vi "quick_plot_for_one_channel.vi"() -> ()   [LabVIEW 2018]
uses:
  <vilib>/Utility/file.llb/Read Delimited Spreadsheet (string).vi
panel:
  in  "End Time":timestamp
  in  "Start Time":timestamp
  in  "Property":T1(ring)
  out "Graph":cluster{timestamp[], dbl[]}(graph)
  out "all rows":string[][](array[string])
  # "As of 16-01-2020 columns are:\n[0]: on/off\n[1]: status\n[2]: channel name\n[3]: crate\n[4]: card type\n[5]: card\n[6]: channel\n[7]: vswmax\n[8]: vmon\n[9]: vset\n[10]: imon\n[11]: iset\n[12]: timestamp\n[13: flag"
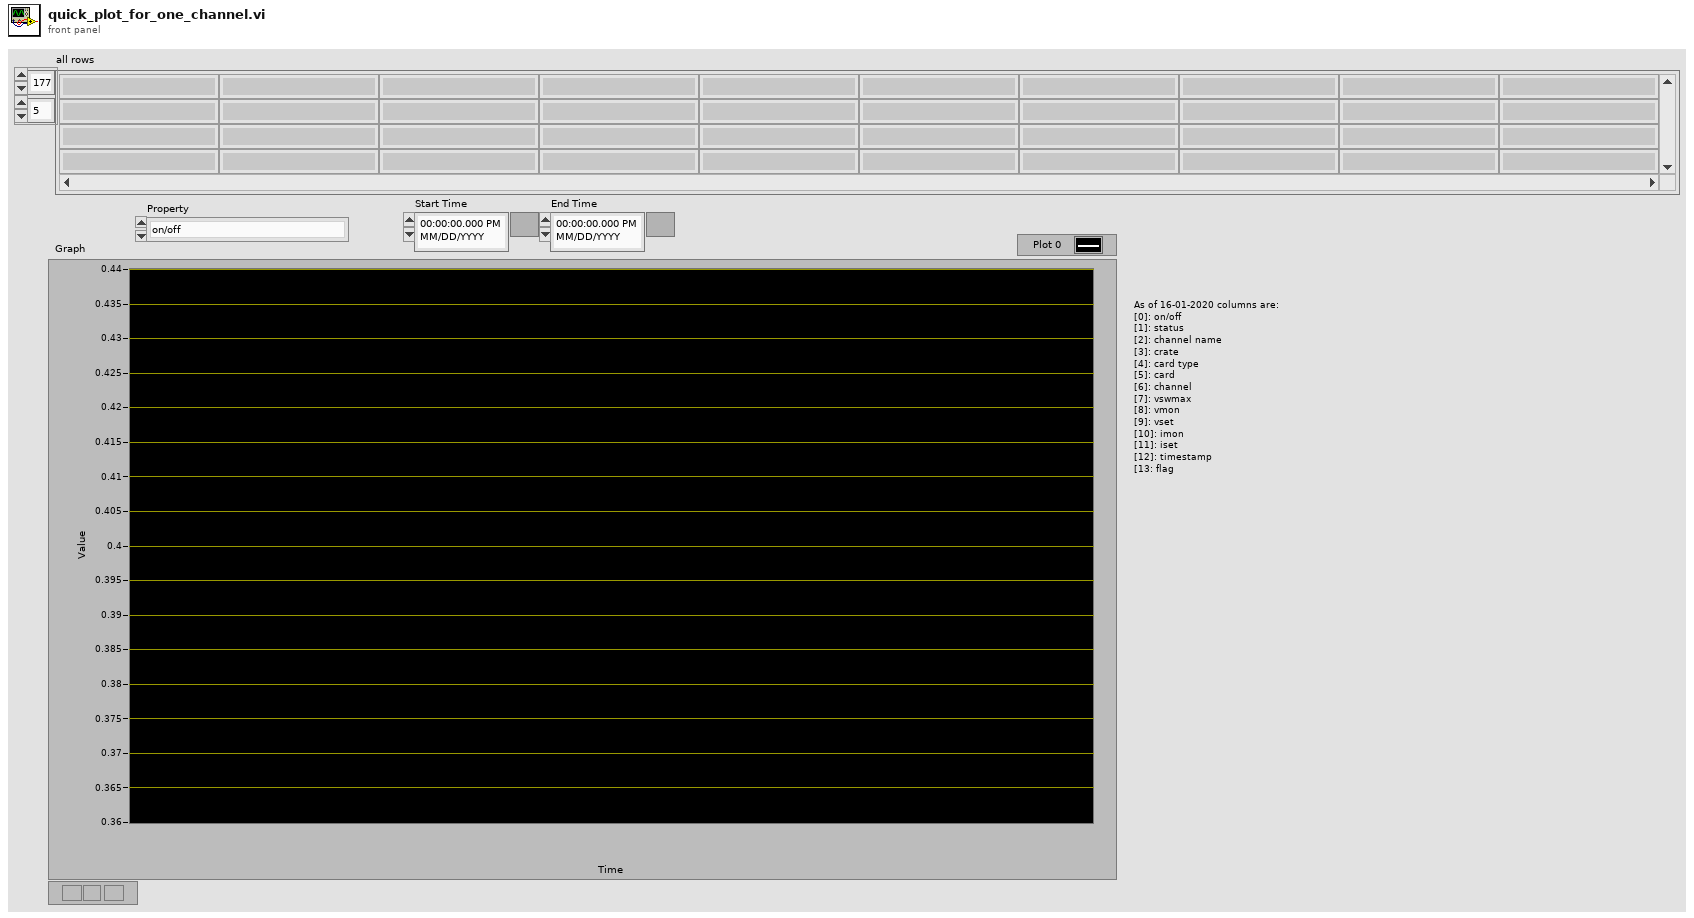
[diagram p1: front panel]
types:
  T1 = enum16{"on/off", "status", "channel_name", "crate_num", "card_type", "card", "channel", "Vswmax", "Vmon", "Vset", "Imon", "Imax", "Timestamp", "Flagged"}
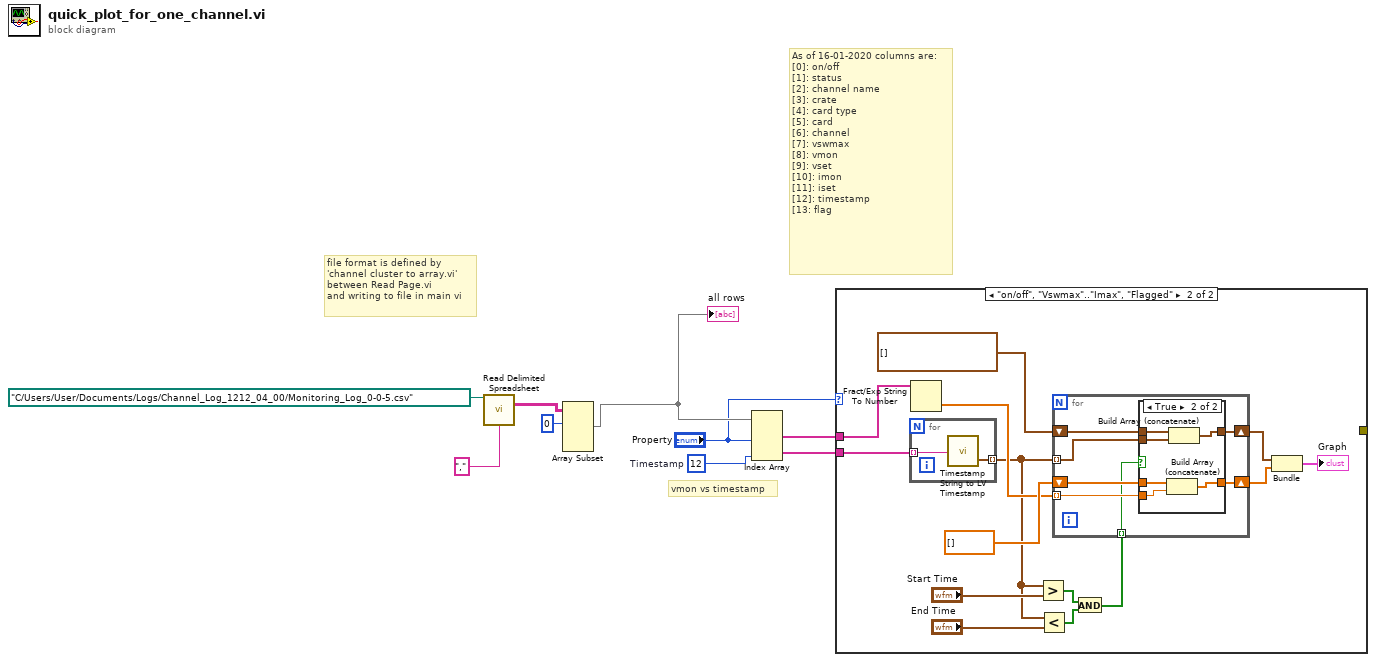
[diagram p0: block diagram]
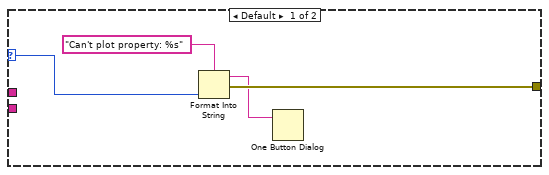
[diagram p2: hidden frame]
diagram:
  w7 = 12  # Timestamp
  # "vmon vs timestamp"
  # "As of 16-01-2020 columns are:\n[0]: on/off\n[1]: status\n[2]: channel name\n[3]: crate\n[4]: card type\n[5]: card\n[6]: channel\n[7]: vswmax\n[8]: vmon\n[9]: vset\n[10]: imon\n[11]: iset\n[12]: timestamp\n[13: flag"
  # "file format is defined by\n'channel cluster to array.vi'\nbetween Read Page.vi\nand writing to file in main vi"
  n1 = call-poly <vilib>:"Read Delimited Spreadsheet.vi"("file path (dialog if empty)"=path "C:/Users/User/Documents/Logs/Channel_Log_1212_04_00/Monitoring_Log_0-0-5.csv", "delimiter (\\t)"="," ("delimiter (\\t)")) -> ("all rows"=w4:string[][])  [unwired: 8 in, 5 out]
  n2 = Array Subset(array=w4, index (row)=0 ("index")) -> (w3:string[][])  [unwired: 3 in]
  "all rows" <- w3
  n3 = Index Array(array=w3, index (col) #1="Property", index (col) #2=w7) -> (element #1=w6:string[], element #2=w5:string[])  [unwired: 2 in]
  n4 = case shown="\"on/off\", \"Vswmax\"..\"Imax\", \"Flagged\"" "Property" {
    selector: "Property" -> [w10 _]
    tunnel: w6 -> [_ w27]
    tunnel: w5 -> [_ w26]
    tunnel: [w12 _] -> _
    frame Default {
      n5 = Format Into String(format string="Can't plot property: %s", w10) -> (resulting string=w11:string, error out=w12:errorcluster)  [unwired: 2 in]
      n6 = One Button Dialog(message=w11) -> ()  [unwired: 1 in, 1 out]
    }
    frame "on/off", "Vswmax".."Imax", "Flagged" {
      n7 = for {
        tunnel: w26 -> [w44] mode=indexing
        tunnel: [w43] -> w14 mode=indexing
        n8 = call "Timestamp String to LV Timestamp.vi"("Timestamp String"=w44) -> ("Timestamp"=w43:timestamp)  [unwired: 1 out]
      }
      n9 = Fract/Exp String To Number(string=w27) -> (number=w23:dbl[])  [unwired: 3 in, 1 out]
      n10 = Greater?(x=w14, y="Start Time") -> (0:w17:bool[])
      n11 = Less?(x=w14, y="End Time") -> (x < y?=w16:bool[])
      n12 = And(x=w17, y=w16) -> (x .and. y?=w15:bool[])
      n13 = for {
        shift-right: [w31] -> w22
        shift-left: timestamp[] [] -> [w32]
        shift-right: [w29] -> w21
        shift-left: dbl[] [] ("number") -> [w30]
        tunnel: w23 -> [w34] mode=indexing
        tunnel: w14 -> [w33] mode=indexing
        tunnel: w15 -> [w28] mode=indexing
        n14 = case shown="True" w28 {
          tunnel: w34 -> [_ w39]
          tunnel: w33 -> [_ w42]
          tunnel: w32 -> [w36 w41]
          tunnel: [w36 w40] -> w31
          tunnel: w30 -> [w35 w38]
          tunnel: [w35 w37] -> w29
          frame False {
          }
          frame True {
            n15 = Build Array (concatenate)(w38, w39) -> (w37:dbl[])
            n16 = Build Array (concatenate)(w41, w42) -> (w40:timestamp[])
          }
        }
      }
      n17 = Bundle(w22, "number"=w21) -> (→"Graph":cluster{timestamp[], "number":dbl[]})  [unwired: 1 in]
    }
  }
